vi "Create or Add Phrase or Paragraph with Images.vi"(0 "Leading":sgl=12.0, 1 "Phrase or paragraph":T2, 2 "Text zone (points)":cluster{"widht":sgl, "height":sgl}={"widht"=612.0, "height"=792.0}, 3 "Image offsetY":sgl, 5 "Phrase refnum IN":refnum<k24>, 7 "Paragraph refnum IN":refnum<k24>, 9 "Text":string, 11 "error in (no error)":errorcluster, 12 "Font refnum":refnum<k24>, 13 "Paragraph indentation (points)":T3, 14 "Image to Add refnum [ ]":T1) -> (4 "Leading duplicate":sgl=12.0, 6 "Phrase refnum OUT":refnum<k24>, 8 "Paragraph refnum OUT":refnum<k24>, 10 "Image?":bool, 15 "error out":errorcluster)   [LabVIEW 2013]
doc: "Version 1.0\nDeveloped by Jean-Marc Simard\nCopyright © 2010, Exaprom Inc.\nAll rights reserved.\nLicense: BSD\n\nWith iTextSharp 4.1.6 (http://itextsharp.sourceforge.net)\nunder Mozilla Public License Version 1.1\n(http://www.mozilla.org/MPL/MPL-1.1.html)"
uses:
  C:/Users/MaxCorp/Documents/GitHub/TopView/DLL/itextsharp.dll
  DLL/itextsharp.dll
  Controls/Paragraph indentation.ctl
  Controls/Phrase or paragraph.ctl
  Controls/Image to Add refnum [ ].ctl
  Controls/Text element type.ctl
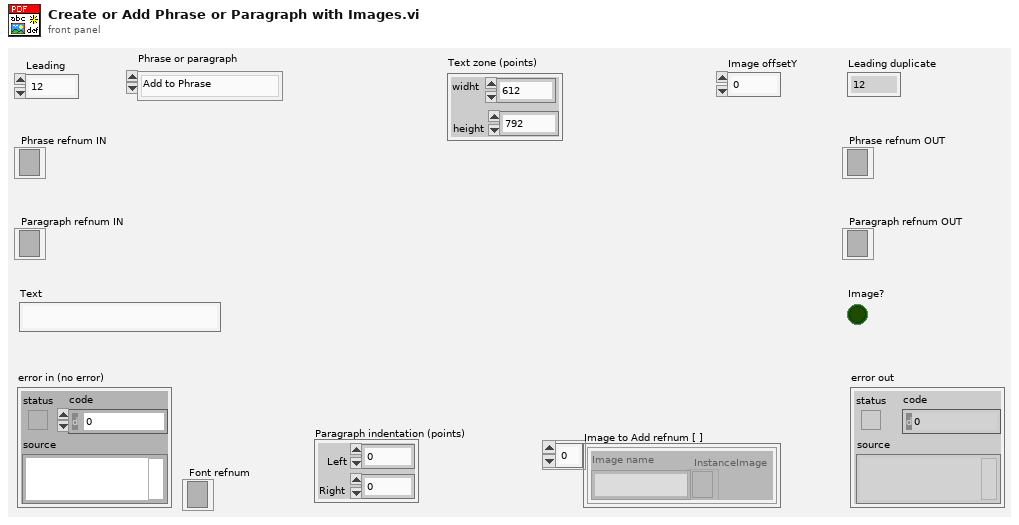
[diagram p1: front panel]
types:
  T1 = typedef "Image to Add refnum [ ].ctl" = cluster{"Image name":string, "InstanceImage":refnum<k24>}[]
  T2 = typedef "Phrase or paragraph.ctl" = enum16{"Add to Phrase", "Add to Paragraph", "Create Phrase", "Create Paragraph"}
  T3 = typedef "Paragraph indentation.ctl" = cluster{"Left":sgl, "Right":sgl}
  T4 = typedef "Text element type.ctl" = enum16{"Text", "Image", "Not a valid image", "Link"}
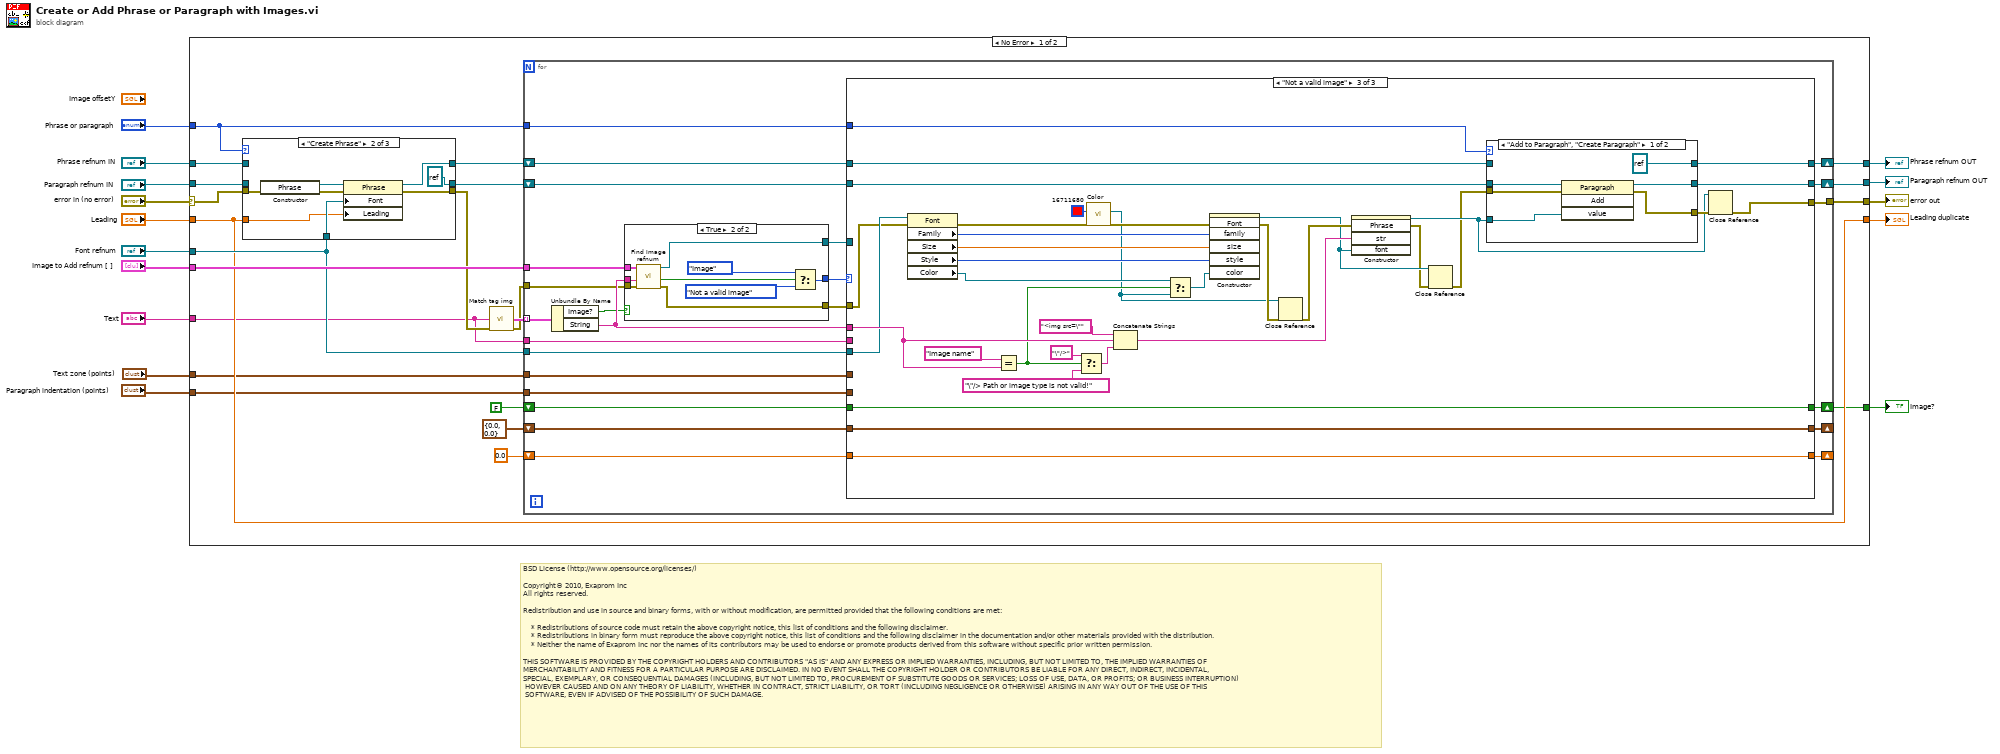
[diagram p0: block diagram]
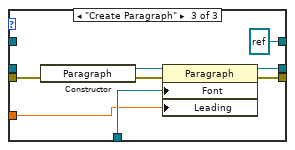
[diagram p3: hidden frame]
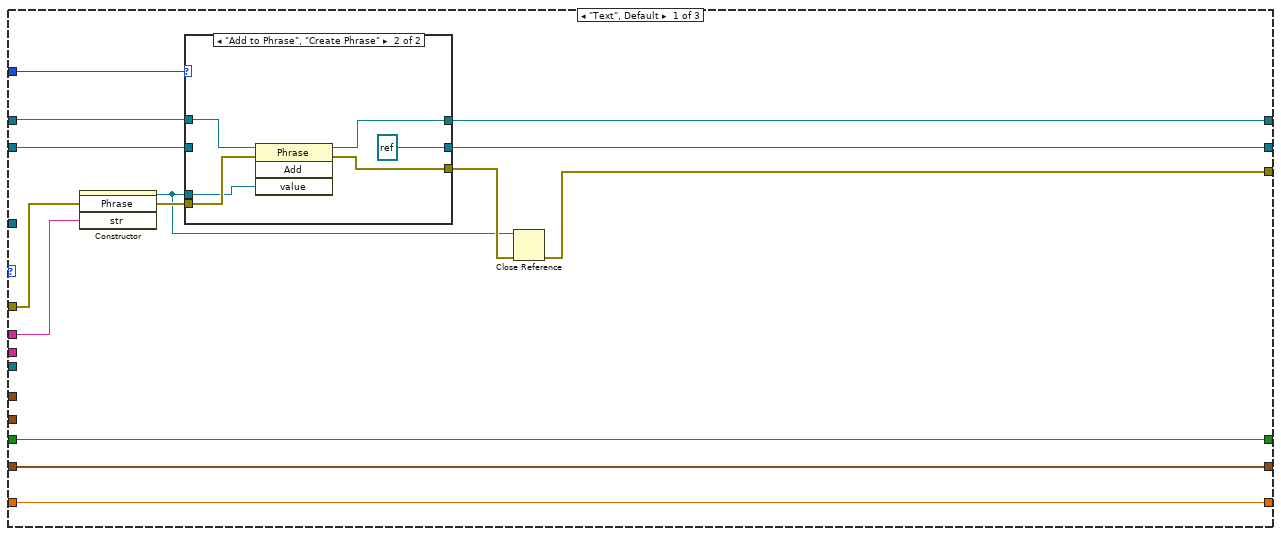
[diagram p4: hidden frame]
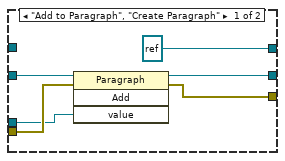
[diagram p5: hidden frame]
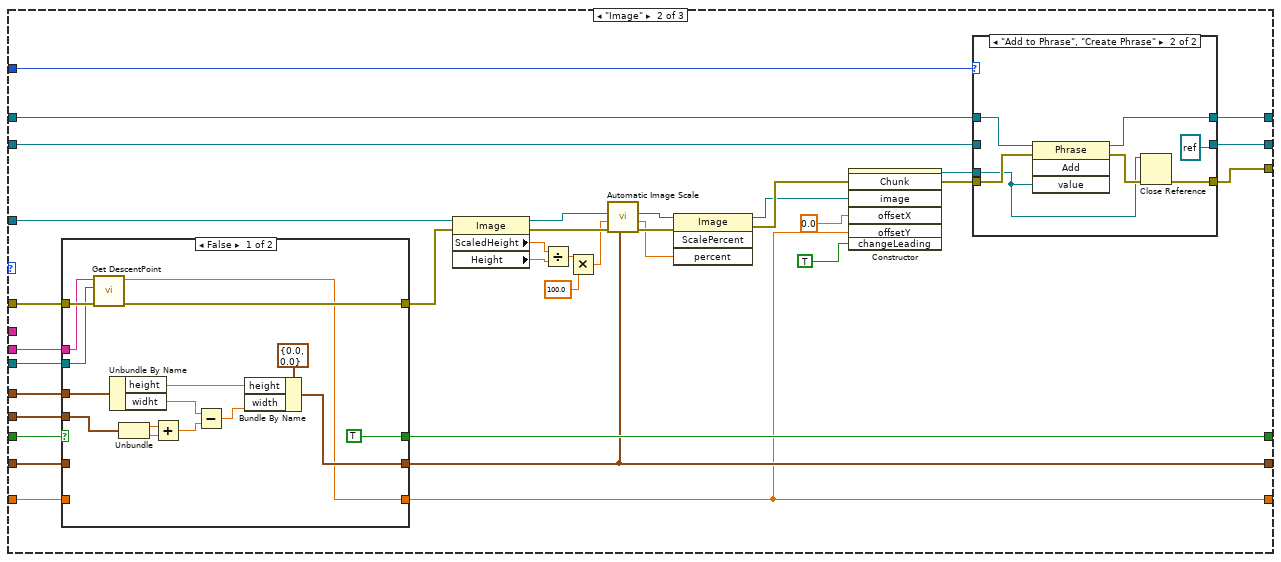
[diagram p6: hidden frame]
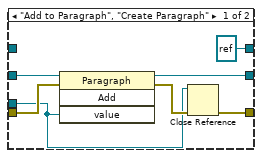
[diagram p8: hidden frame]
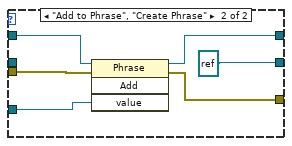
[diagram p9: hidden frame]
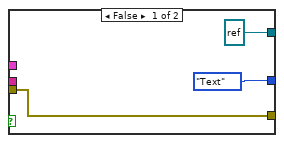
[diagram p10: hidden frame]
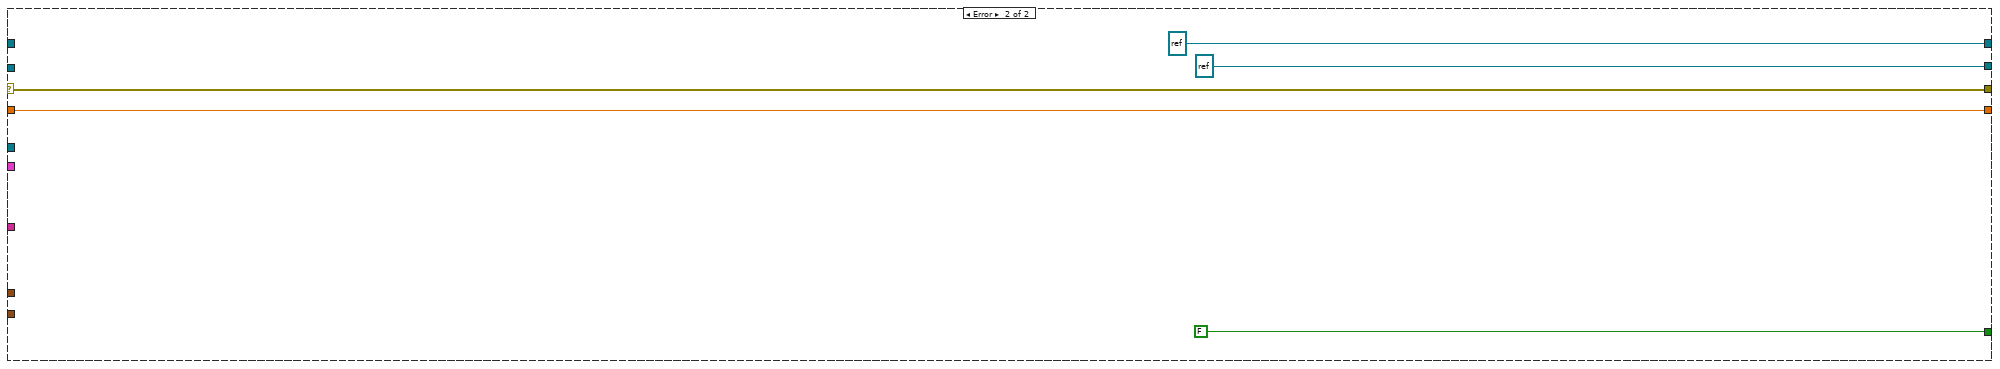
[diagram p11: hidden frame]
diagram:
  # "BSD License (http://www.opensource.org/licenses/)\n\nCopyright© 2010, Exaprom Inc\nAll rights reserved.\n\nRedistribution and use in source and binary forms, with or without modification, are permitted provided that the following conditions are met:\n\n    * Redistributions of source code must retain the above copyright notice, this list of conditions and the following disclaimer.\n    * Redistributions in binary form must reproduce the above copyright notice, this list of conditions and the following disclaimer in the documentation and/or other materials provided with the distribution.\n    * Neither the name of Exaprom Inc nor the names of its contributors may be used to endorse or promote products derived from this software without specific prior written permission.\n\nTHIS SOFTWARE IS PROVIDED BY THE COPYRIGHT HOLDERS AND CONTRIBUTORS \"AS IS\" AND ANY EXPRESS OR IMPLIED WARRANTIES, INCLUDING, BUT NOT LIMITED TO, THE IMPLIED WARRANTIES OF \nMERCHANTABILITY AND FITNESS FOR A PARTICULAR PURPOSE ARE DISCLAIMED. IN NO EVENT SHALL THE COPYRIGHT HOLDER OR CONTRIBUTORS BE LIABLE FOR ANY DIRECT, INDIRECT, INCIDENTAL,\nSPECIAL, EXEMPLARY, OR CONSEQUENTIAL DAMAGES (INCLUDING, BUT NOT LIMITED TO, PROCUREMENT OF SUBSTITUTE GOODS OR SERVICES; LOSS OF USE, DATA, OR PROFITS; OR BUSINESS INTERRUPTION)\n HOWEVER CAUSED AND ON ANY THEORY OF LIABILITY, WHETHER IN CONTRACT, STRICT LIABILITY, OR TORT (INCLUDING NEGLIGENCE OR OTHERWISE) ARISING IN ANY WAY OUT OF THE USE OF THIS\n SOFTWARE, EVEN IF ADVISED OF THE POSSIBILITY OF SUCH DAMAGE."
  n1 = case shown="No Error" "error in (no error)" {
    selector: "error in (no error)" -> [w30 w239]
    tunnel: "Image to Add refnum [ ]" -> [w37 _]
    tunnel: "Text" -> [w18 _]
    tunnel: [w27 refnum<k24> refnum ("new reference")] -> w5
    tunnel: "Leading" -> [w25 w236]
    tunnel: "Font refnum" -> [w29 _]
    tunnel: [w26 w239] -> w11
    tunnel: "Text zone (points)" -> [w19 _]
    tunnel: "Paragraph indentation (points)" -> [w20 _]
    tunnel: "Phrase or paragraph" -> [w31 _]
    tunnel: [w28 refnum<k24> refnum ("new reference")] -> w6
    tunnel: [w25 w236] -> w8
    tunnel: "Phrase refnum IN" -> [w22 _]
    tunnel: "Paragraph refnum IN" -> [w21 _]
    tunnel: [w16 FALSE] -> w2
    frame No Error {
      n2 = case shown="\"Create Phrase\"" w31 {
        tunnel: [w39 refnum<k24> refnum ("new reference") w54] -> w34
        tunnel: [w38 w46 w53] -> w33
        tunnel: w29 -> [_ w45 w52]
        tunnel: [w40 w44 refnum<k24> refnum ("new reference")] -> w32
        tunnel: w30 -> [w38 w42 w50]
        tunnel: w25 -> [_ w41 w49]
        tunnel: w22 -> [w40 _ _]
        tunnel: w21 -> [w39 _ _]
        frame "Add to Phrase", "Add to Paragraph" {
        }
        frame "Create Phrase" {
          n3 = constructor class="Phrase"(error in=w42) -> (reference out=w48:refnum<k24>, error out=w47:errorcluster)  [unwired: 2 in, 1 out]
          n4 = property class="Phrase"(reference=w48, error in=w47, "Font"=w45, "Leading"=w41) -> (reference out=w44:refnum<k24>, error out=w46:errorcluster)
        }
        frame "Create Paragraph" {
          n5 = constructor class="Paragraph"(error in=w50) -> (reference out=w55:refnum<k24>, error out=w56:errorcluster)  [unwired: 2 in, 1 out]
          n6 = property class="Paragraph"(reference=w55, error in=w56, "Font"=w52, "Leading"=w49) -> (reference out=w54:refnum<k24>, error out=w53:errorcluster)
        }
      }
      n7 = call "Match tag img.vi"("String"=w18, "error in (no error)"=w33) -> ("Text [ ]"=w36:cluster{"String":string, "Image?":bool}[], "error out"=w35:errorcluster)  [unwired: 12 out]
      n8 = for {
        tunnel: w36 -> [w80] mode=indexing
        shift-right: [w69] -> w27
        shift-left: w34 -> [w79]
        tunnel: w37 -> [w74]
        tunnel: w35 -> [w73]
        tunnel: [w70] -> w26
        tunnel: w20 -> [w78]
        shift-right: [w68] -> w28
        shift-left: w32 -> [w76]
        tunnel: w31 -> [w77]
        tunnel: w29 -> [w66]
        shift-right: [w61] -> w16
        shift-left: FALSE -> [w62]
        shift-right: [w58] -> _
        shift-left: sgl 0.0 ("GetDescentPoint") -> [w57]
        tunnel: w19 -> [w65]
        tunnel: w18 -> [w64]
        shift-right: [w60] -> _
        shift-left: cluster{"width":sgl, "height":sgl} {"width"=0.0, "height"=0.0} ("Box") -> [w59]
        n9 = Unbundle By Name(w80) -> ("Image?"=w67:bool, "String"=w75:string)
        n10 = case shown="True" w67 {
          tunnel: w75 -> [_ w234]
          tunnel: w74 -> [_ w233]
          tunnel: [refnum<k24> refnum ("InstanceImage refnum") w232] -> w72
          tunnel: w73 -> [w224 w231]
          tunnel: [w224 w228] -> w63
          tunnel: [Text_element_type."Text" ("Text element type") w226] -> w71
          frame False {
          }
          frame True {
            n11 = call "Find Image refnum.vi"("error in (no error)"=w231, "Image Name"=w234, "Image to Add refnum [ ]"=w233) -> ("error out"=w228:errorcluster, "Find Image?"=w230:bool, "InstanceImage refnum"=w232:refnum<k24>)  [unwired: 6 out]
            n12 = Select(t=Text_element_type."Image" ("Text element type"), s=w230, f=Text_element_type."Not a valid image" ("Text element type")) -> (s? t:f=w226:T4)
          }
        }
        n13 = case shown="\"Not a valid image\"" w71 {
          tunnel: [w92 w139 w201] -> w69
          tunnel: w79 -> [w88 w140 w194]
          tunnel: w63 -> [w93 w116 w192]
          tunnel: [w86 w137 w197] -> w70
          tunnel: w78 -> [_ w118 _]
          tunnel: w77 -> [w90 w124 w198]
          tunnel: w76 -> [w89 w126 w195]
          tunnel: [w91 w125 w200] -> w68
          tunnel: w75 -> [w85 _ w210]
          tunnel: w66 -> [_ w114 w204]
          tunnel: w72 -> [_ w119 _]
          tunnel: w65 -> [_ w117 _]
          tunnel: w64 -> [_ w113 _]
          tunnel: w62 -> [w84 w112 w178]
          tunnel: [w84 w111 w178] -> w61
          tunnel: [w83 w109 w177] -> w60
          tunnel: w59 -> [w83 w110 w177]
          tunnel: [w82 w107 w176] -> w58
          tunnel: w57 -> [w82 w108 w176]
          frame "Text", Default {
            n14 = constructor class="Phrase"(error in=w93, "str"=w85) -> (reference out=w81:refnum<k24>, error out=w94:errorcluster)  [unwired: 2 in, 2 out]
            n15 = case shown="\"Add to Phrase\", \"Create Phrase\"" w90 {
              tunnel: w88 -> [w100 _]
              tunnel: w94 -> [w99 w106]
              tunnel: w81 -> [w98 w105]
              tunnel: [w95 w101] -> w87
              tunnel: [w97 refnum<k24> refnum ("new reference")] -> w92
              tunnel: w89 -> [_ w104]
              tunnel: [refnum<k24> refnum ("new reference") w103] -> w91
              frame "Add to Paragraph", "Create Paragraph" {
                n16 = invoke class="Paragraph" method="Add"(reference=w100, error in=w99, "value"=w98) -> (reference out=w97:refnum<k24>, error out=w95:errorcluster)  [unwired: 1 in, 2 out]
              }
              frame "Add to Phrase", "Create Phrase" {
                n17 = invoke class="Phrase" method="Add"(reference=w104, error in=w106, "value"=w105) -> (reference out=w103:refnum<k24>, error out=w101:errorcluster)  [unwired: 1 in, 2 out]
              }
            }
            n18 = Close Reference(reference=w81, error in (no error)=w87) -> (error out=w86:errorcluster)
          }
          frame "Image" {
            n19 = case shown="False" w112 {
              selector: w112 -> [_ w160]
              tunnel: w118 -> [w152 _]
              tunnel: w117 -> [w151 _]
              tunnel: [w150 w161] -> w115
              tunnel: w116 -> [w149 w161]
              tunnel: w114 -> [w148 _]
              tunnel: w113 -> [w147 _]
              tunnel: [TRUE w160] -> w111
              tunnel: [w145 w159] -> w109
              tunnel: w110 -> [_ w159]
              tunnel: [w144 w158] -> w107
              tunnel: w108 -> [_ w158]
              frame False {
                n20 = call "Get DescentPoint.vi"("error in (no error)"=w149, "Font refnum"=w148, "String"=w147) -> ("error out"=w150:errorcluster, "DescentPoint"=w144:sgl)  [unwired: 1 in, 6 out]
                n21 = Unbundle By Name(w151) -> ("height"=w143:sgl, "widht"=w142:sgl)
                n22 = Unbundle(w152) -> ("Left"=w157:sgl, "Right"=w156:sgl)
                n23 = Add(x=w157, y=w156) -> (x+y=w155:sgl)
                n24 = Subtract(x=w142, y=w155) -> (x-y=w154:sgl)
                n25 = Bundle By Name(cluster=cluster{"width":sgl, "height":sgl} {"width"=0.0, "height"=0.0} ("Box"), "height"=w143, "width"=w154) -> (w145:cluster{"width":sgl, "height":sgl})
              }
              frame True {
              }
            }
            n26 = property class="Image"(reference=w119, error in=w115) -> (reference out=w134:refnum<k24>, error out=w133:errorcluster, "ScaledHeight"=w135:sgl, "Height"=w136:sgl)
            n27 = Divide(x=w135, y=w136) -> (x/y=w132:sgl)
            n28 = Multiply(x=w132, y=sgl 100.0) -> (x*y=w130:sgl)
            n29 = call "Automatic Image Scale.vi"("Box"=w109, "error in (no error)"=w133, "Scale percent IN"=w130, "GetInstanceImage IN"=w134) -> ("error out"=w128:errorcluster, "Scale percent OUT"=w127:sgl, "GetInstanceImage OUT"=w129:refnum<k24>)  [unwired: 2 in, 3 out]
            n30 = invoke class="Image" method="ScalePercent"(reference=w129, error in=w128, "percent"=w127) -> (reference out=w120:refnum<k24>, error out=w121:errorcluster)  [unwired: 1 in, 2 out]
            n31 = constructor class="Chunk"(error in=w121, "image"=w120, "offsetX"=sgl 0.0, "offsetY"=w107, "changeLeading"=TRUE) -> (reference out=w138:refnum<k24>, error out=w141:errorcluster)  [unwired: 2 in, 5 out]
            n32 = case shown="\"Add to Phrase\", \"Create Phrase\"" w124 {
              tunnel: w141 -> [w168 w175]
              tunnel: w140 -> [w167 _]
              tunnel: [w166 refnum<k24> refnum ("new reference")] -> w139
              tunnel: w138 -> [w164 w173]
              tunnel: [w163 w172] -> w137
              tunnel: w126 -> [_ w171]
              tunnel: [refnum<k24> refnum ("new reference") w170] -> w125
              frame "Add to Paragraph", "Create Paragraph" {
                n33 = invoke class="Paragraph" method="Add"(reference=w167, error in=w168, "value"=w164) -> (reference out=w166:refnum<k24>, error out=w165:errorcluster)  [unwired: 1 in, 2 out]
                n34 = Close Reference(reference=w164, error in (no error)=w165) -> (error out=w163:errorcluster)
              }
              frame "Add to Phrase", "Create Phrase" {
                n35 = invoke class="Phrase" method="Add"(reference=w171, error in=w175, "value"=w173) -> (reference out=w170:refnum<k24>, error out=w174:errorcluster)  [unwired: 1 in, 2 out]
                n36 = Close Reference(reference=w173, error in (no error)=w174) -> (error out=w172:errorcluster)
              }
            }
          }
          frame "Not a valid image" {
            n37 = property class="Font"(reference=w204, error in=w192) -> (error out=w203:errorcluster, "Family"=w190:i32, "Size"=w189:sgl, "Style"=w188:i32, "Color"=w180:refnum<k24>)  [unwired: 1 out]
            n38 = Equal?(x="Image name", y=w210) -> (x = y?=w181:bool)
            n39 = Select(t="\"/>", s=w181, f="\"/> Path or image type is not valid!") -> (s? t:f=w207:string)
            n40 = call "Color.vi"("error in (no error)"=w203, "Color"=u32 16711680) -> ("error out"=w191:errorcluster, "Color"=w179:refnum<k24>)  [unwired: 8 out]
            n41 = Concatenate Strings("<img src=\"", w210, w207) -> (w199:string)
            n42 = Select(t=w180, s=w181, f=w179) -> (s? t:f=w182:refnum<k24>)
            n43 = constructor class="Font"(error in=w191, "family"=w190, "size"=w189, "style"=w188, "color"=w182) -> (reference out=w185:refnum<k24>, error out=w187:errorcluster)  [unwired: 2 in, 5 out]
            n44 = Close Reference(reference=w179, error in (no error)=w187) -> (error out=w186:errorcluster)
            n45 = constructor class="Phrase"(error in=w186, "str"=w199, "font"=w185) -> (reference out=w193:refnum<k24>, error out=w184:errorcluster)  [unwired: 2 in, 3 out]
            n46 = Close Reference(reference=w185, error in (no error)=w184) -> (error out=w183:errorcluster)
            n47 = case shown="\"Add to Paragraph\", \"Create Paragraph\"" w198 {
              tunnel: w183 -> [w216 w222]
              tunnel: w194 -> [w215 _]
              tunnel: [w212 refnum<k24> refnum ("new reference")] -> w201
              tunnel: w193 -> [w214 w221]
              tunnel: [w211 w218] -> w196
              tunnel: w195 -> [_ w220]
              tunnel: [refnum<k24> refnum ("new reference") w217] -> w200
              frame "Add to Paragraph", "Create Paragraph" {
                n48 = invoke class="Paragraph" method="Add"(reference=w215, error in=w216, "value"=w214) -> (reference out=w212:refnum<k24>, error out=w211:errorcluster)  [unwired: 1 in, 2 out]
              }
              frame "Add to Phrase", "Create Phrase" {
                n49 = invoke class="Phrase" method="Add"(reference=w220, error in=w222, "value"=w221) -> (reference out=w217:refnum<k24>, error out=w218:errorcluster)  [unwired: 1 in, 2 out]
              }
            }
            n50 = Close Reference(reference=w193, error in (no error)=w196) -> (error out=w197:errorcluster)
          }
        }
      }
    }
    frame Error {
    }
  }
  "error out" <- w11
  "Paragraph refnum OUT" <- w5
  "Phrase refnum OUT" <- w6
  "Leading duplicate" <- w8
  "Image?" <- w2
